vi "MainRIOJuan.vi"() -> ()   [LabVIEW 2019]
uses:
  RIOData--cluster.ctl
  Acelerometer data--cluster.ctl
  <vilib>/PantherLAB/Firebase API/PantherLAB_lib_Filtering Parameters--cluster.ctl
  a087fea8-a487-4c1c-8a8b-15f205e78756.vi
  c90b4970-0cb1-4ed8-a3e8-abf7f56642d0.vi
  079ee137-338a-4224-8d27-3950f07d8dd5.vi
  <vilib>/JDP Science/JSONtext/JSON text to Variant.vi
  <vilib>/JDP Science/JSONtext/LVClass Serializer/JSONtext LVClass Serializer.lvclass
  <vilib>/PantherLAB/Firebase API/PantherLAB_lib_firebase.lvclass
  Shared.lvlib
  <vilib>/JDP Science/JSONtext/JSONtext.lvlib
panel:
  in  "Get All":bool
  in  "Get5":bool
  out "JSON String":string
  in  "Get Newest":bool
  in  "Delete":bool
  in  "Password":string
  in  "Email":string
  in  "Log In":bool
  in  "Sign In":bool
  out "Newest":T1
  out "Data out":T1[](array[typedef])
  out "My RIO Acelerometer":T2(graph)
  # "To add an authenticated user\nto your Real Time Database"
  # "If you are already authenticated\nand you want to start using\nyour Database"
  # "Warning:\nThis button will delete all the data\nunder Post EndPoint"
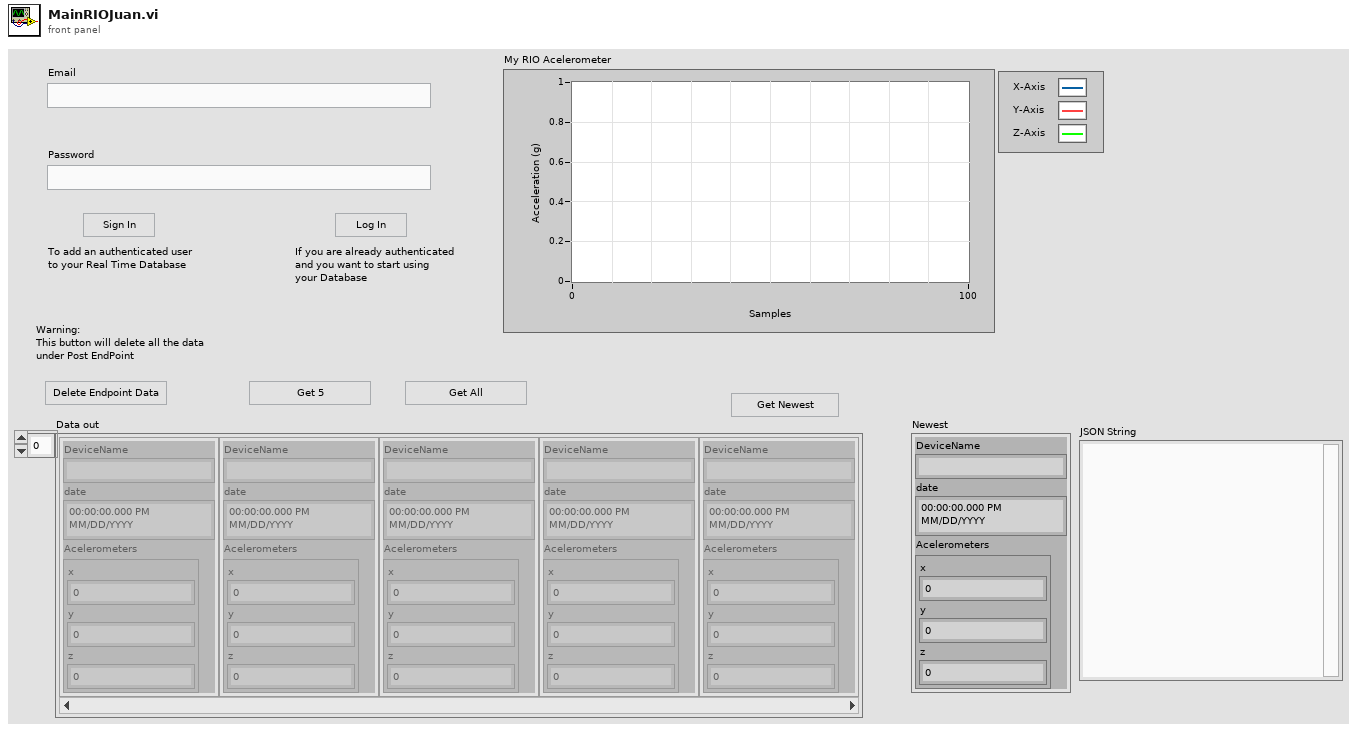
[diagram p1: front panel]
types:
  T1 = typedef "Shared.lvlib/RIOData--cluster.ctl" = cluster{"DeviceName":string, "date":timestamp, "Acelerometers":cluster{"x":dbl, "y":dbl, "z":dbl}}
  T2 = typedef "Shared.lvlib/Acelerometer data--cluster.ctl" = cluster{"X-Axis":dbl, "Y-Axis":dbl, "Z-Axis":dbl}
  T3 = cluster{"Read Access":enum8{"Allowed", "Required", "None"}, "Write Access":enum8{"Allowed", "Required", "None"}}
  T4 = typedef "PantherLAB_lib_firebase.lvclass/PantherLAB_lib_Filtering Parameters--cluster.ctl" = cluster{"Filtering Param":string, "Argument":string}
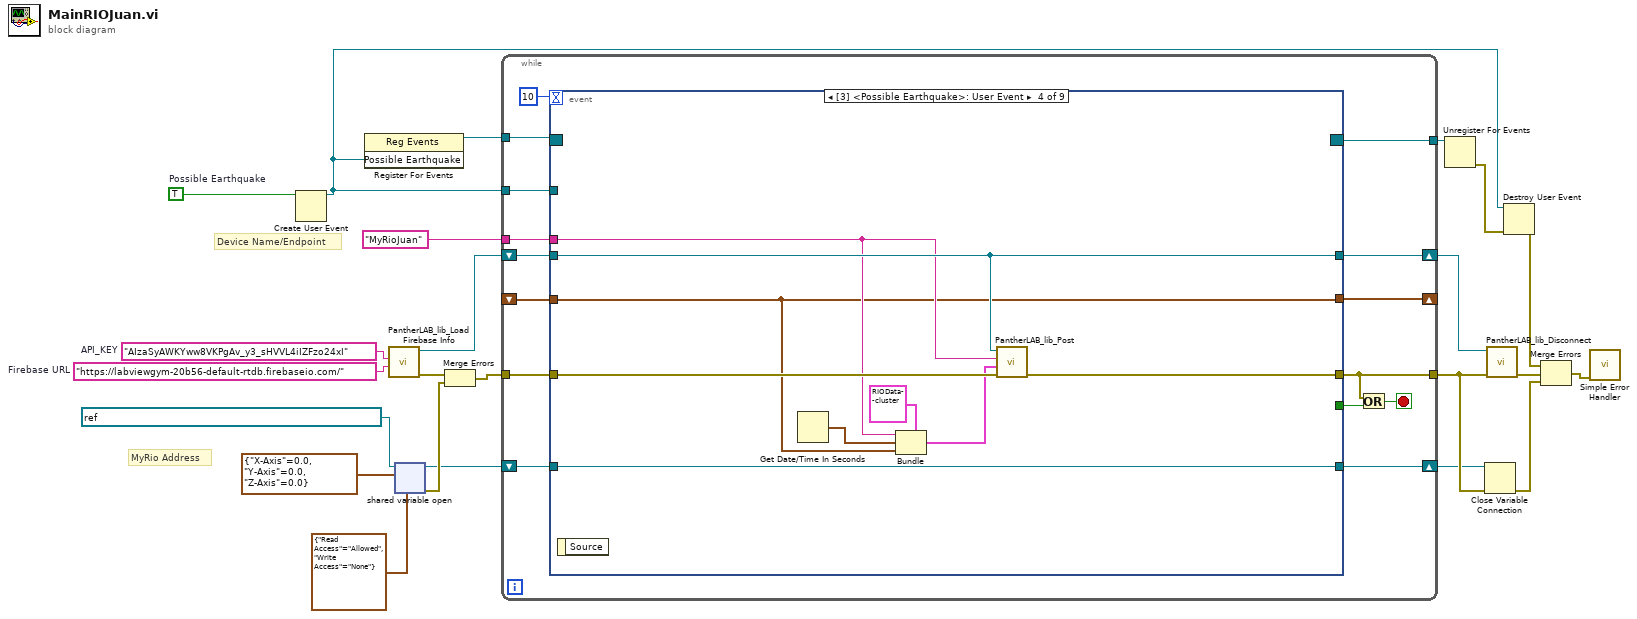
[diagram p0: block diagram]
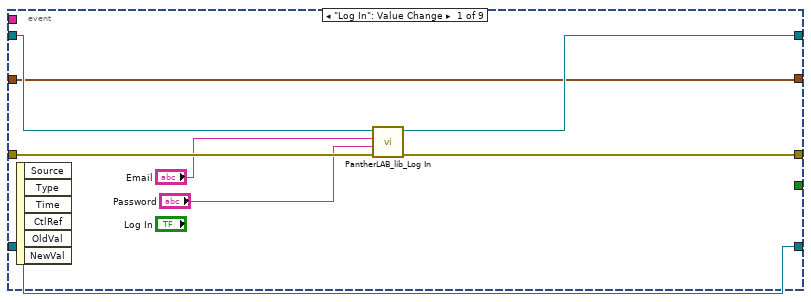
[diagram p2: hidden frame]
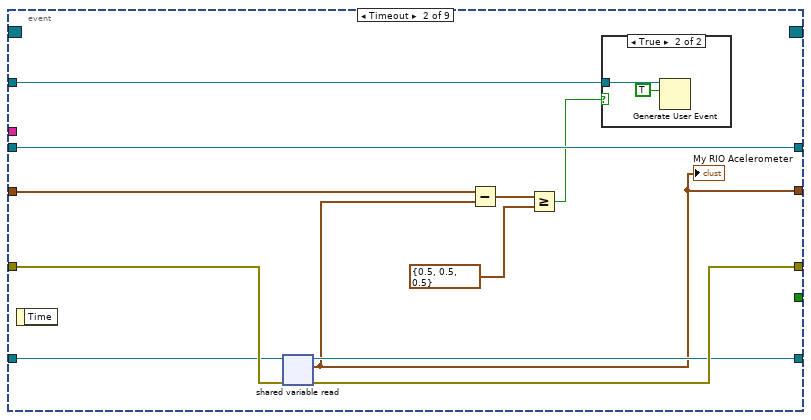
[diagram p3: hidden frame]
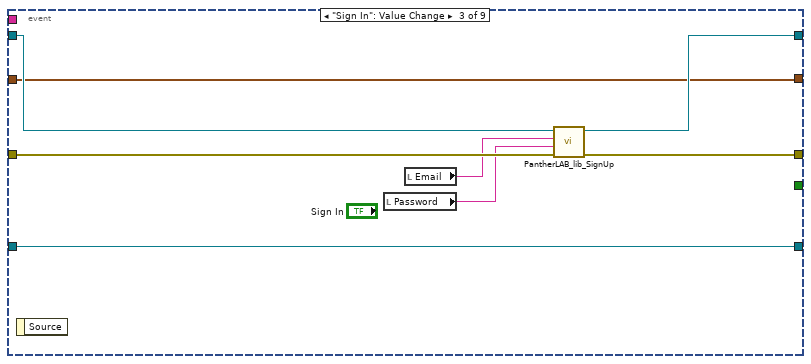
[diagram p5: hidden frame]
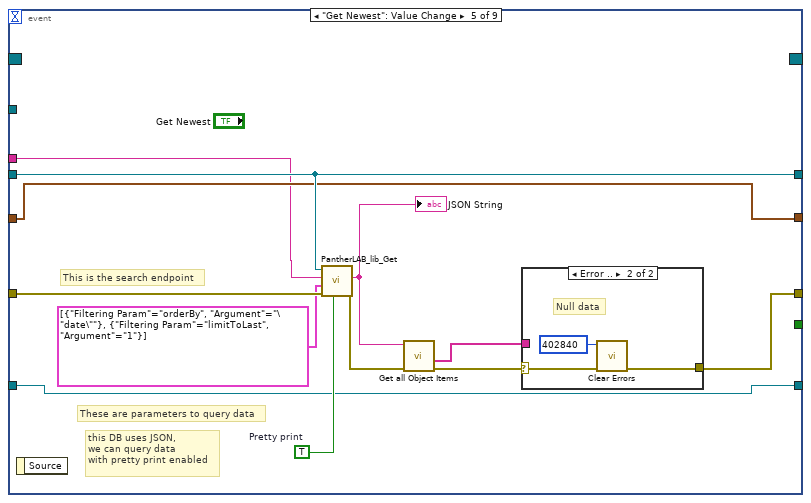
[diagram p6: hidden frame]
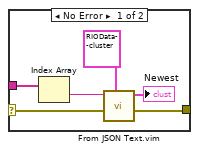
[diagram p7: hidden frame]
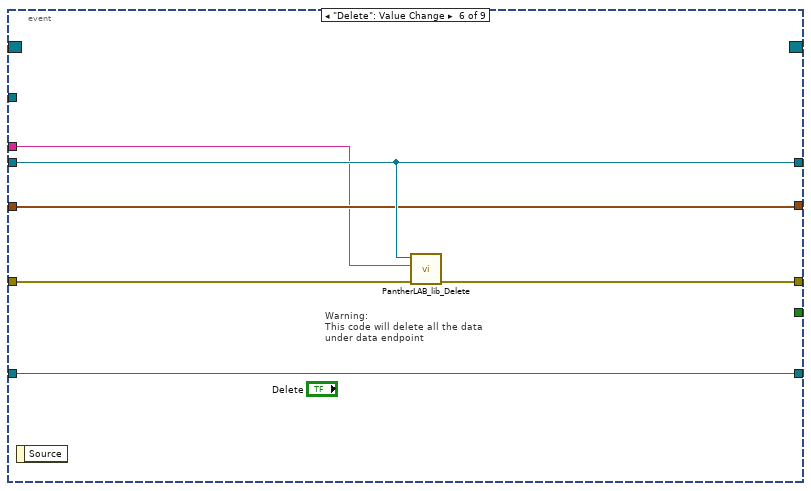
[diagram p8: hidden frame]
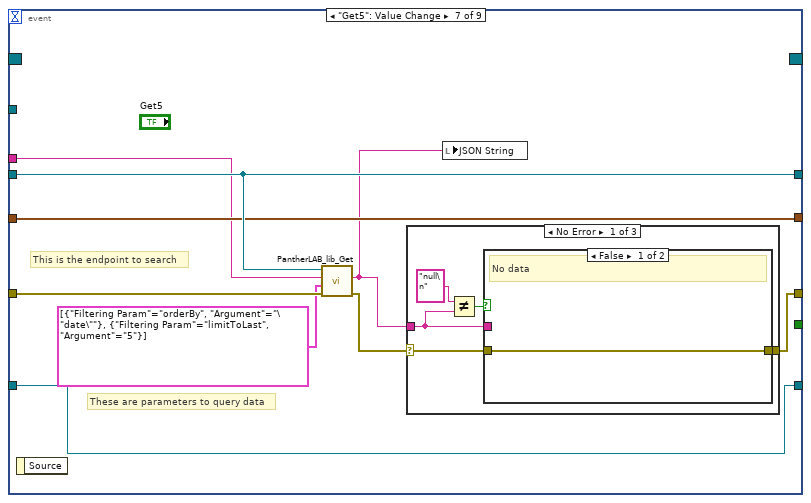
[diagram p9: hidden frame]
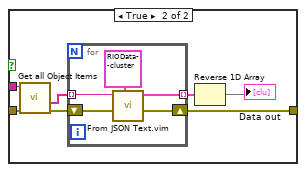
[diagram p10: hidden frame]
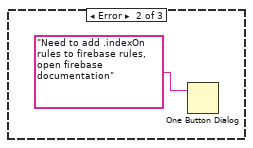
[diagram p11: hidden frame]
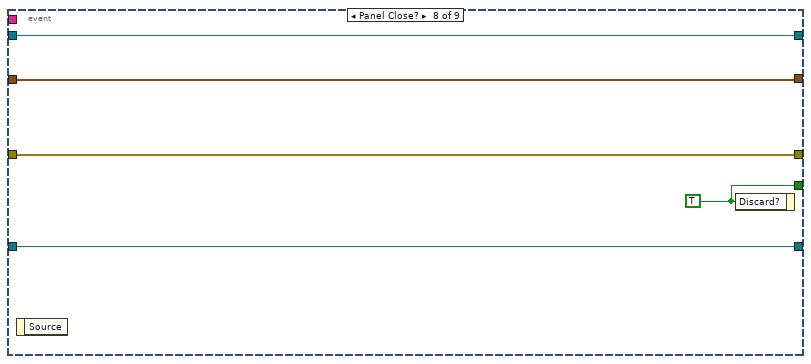
[diagram p13: hidden frame]
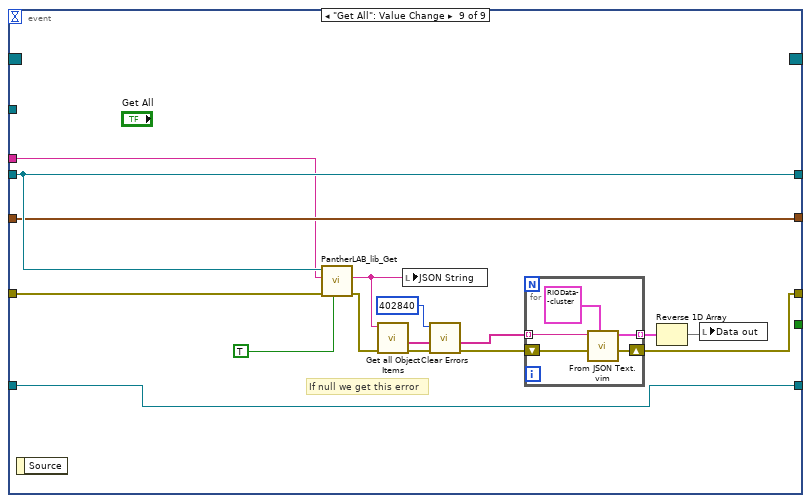
[diagram p14: hidden frame]
diagram:
  w4 = TRUE  # Possible Earthquake
  w9 = "AIzaSyAWKYww8VKPgAv_y3_sHVVL4iIZFzo24xI"  # API_KEY
  w8 = "https://labviewgym-20b56-default-rtdb.firebaseio.com/"  # Firebase URL
  # "MyRio Address"
  # "Device Name/Endpoint"
  n1 = Create User Event(user event datatype=w4) -> (user event=w2:refnum<user-event>)  [unwired: 1 in, 1 out]
  n2 = register-events(w2) -> (reference out=w5:refnum<event-registration>)  [unwired: 2 in, 1 out]
  n3 = call <vilib>:"PantherLAB_lib_Load Firebase Info.vi"("Firebase URL"=w8, "API_KEY"=w9) -> ("error out"=w22:errorcluster, "firebase out"=w10:refnum<class "PantherLAB_lib_firebase.lvclass">)  [unwired: 8 in]
  n4 = shared-variable-open(refnum<k21> "ni.var.psp://192.168.0.227/MyRioLib/AcelerationRIO" ("shared variable refnum in"), T2 {"X-Axis"=0.0, "Y-Axis"=0.0, "Z-Axis"=0.0} ("Acceleration"), T3 {"Read Access"=enum."Allowed", "Write Access"=enum."None"} ("access")) -> (w7:refnum<k21>, w20:errorcluster)  [unwired: 1 in]
  n5 = Merge Errors(w22, w20) -> (w21:errorcluster)
  n6 = while {
    tunnel: w21 -> [w38]
    tunnel: [w37] -> w19
    shift-right: [w33] -> w11
    shift-left: w10 -> [w34]
    shift-right: [w30] -> w6
    shift-left: w7 -> [w31]
    tunnel: w5 -> [w29]
    tunnel: w2 -> [w28]
    shift-right: [w27] -> _
    shift-left: _ -> [w26]
    tunnel: [w25] -> w3
    tunnel: "MyRioJuan" -> [w24]
    stop <- w35 stop-if-true
    n7 = event shown="[3] <Possible Earthquake>: User Event" {
      selector: w29 -> [_ _ _ _ _ _ _ _ _]
      dyn-events: [_ _ _ _ _ _ _ _ _] -> w25
      timeout: 10 -> [_ _ _ _ _ _ _ _ _]
      tunnel: w38 -> [w46 w57 w67 w76 w88 w103 w112 w137 w152]
      tunnel: [w45 w56 w66 w75 w86 w102 w110 w137 w149] -> w37
      tunnel: [_ _ _ _ _ _ _ w135 _] -> w36
      tunnel: w34 -> [w42 w55 w63 w74 w82 w101 w108 w136 w142]
      tunnel: [w41 w55 w62 w74 w82 w101 w108 w136 w142] -> w33
      tunnel: w31 -> [w40 w54 w61 w73 w81 w100 w107 w134 w141]
      tunnel: [w40 w53 w61 w73 w81 w100 w107 w134 w141] -> w30
      tunnel: w28 -> [_ w50 _ _ _ _ _ _ _]
      tunnel: [w39 w48 w60 w68 w80 w99 w106 w133 w140] -> w27
      tunnel: w26 -> [w39 w49 w60 w68 w80 w99 w106 w133 w140]
      tunnel: w24 -> [_ _ _ w71 w79 w98 w105 _ w139]
      event "Log In": Value Change {
        n8 = event-data() -> ()  [unwired: 1 in, 6 out]
        n9 = call-dynamic "PantherLAB_lib_Log In.vi"("error in"=w46, "password"="Password", "email"="Email", "firebase in"=w42) -> ("error out"=w45:errorcluster, "firebase out"=w41:refnum<class "PantherLAB_lib_firebase.lvclass">)  [unwired: 6 in]
      }
      event Timeout {
        n10 = event-data() -> ()  [unwired: 1 in, 1 out]
        n11 = shared-variable-read(w54, w57) -> (w53:refnum<k21>, w56:errorcluster, w48:T2)  [unwired: 1 out]
        "My RIO Acelerometer" <- w48
        n12 = Subtract(x=w49, y=w48) -> (x-y=w52:T2)
        n13 = Greater Or Equal?(x=w52, y=T2 {"X-Axis"=0.5, "Y-Axis"=0.5, "Z-Axis"=0.5} ("x")) -> (x >= y?=w47:bool)
        n14 = case shown="True" w47 {
          tunnel: w50 -> [_ w59]
          frame False {
          }
          frame True {
            n15 = Generate User Event(user event=w59, event data cluster=TRUE ("event data")) -> ()  [unwired: 2 in, 2 out]
          }
        }
      }
      event "Sign In": Value Change {
        n16 = event-data() -> ()  [unwired: 1 in, 1 out]
        n17 = local read "Password"() -> (w65:string)
        n18 = local read "Email"() -> (w64:string)
        n19 = call-dynamic "PantherLAB_lib_SignUp.vi"("error in"=w67, "password"=w65, "email"=w64, "firebase in"=w63) -> ("error out"=w66:errorcluster, "firebase out"=w62:refnum<class "PantherLAB_lib_firebase.lvclass">)  [unwired: 6 in]
      }
      event User Event {
        n20 = event-data() -> ()  [unwired: 1 in, 1 out]
        n21 = Get Date/Time In Seconds() -> (seconds since 1Jan1904=w70:timestamp)
        n22 = Bundle(cluster=T1 {"DeviceName"="", "date"=timestamp(0 s since 1904-01-01), "Acelerometers"={"x"=0.0, "y"=0.0, "z"=0.0}} ("output cluster"), "DeviceName"=w71, "date"=w70, "Acelerometers"=w68) -> (w72:T1)
        n23 = call-dynamic "PantherLAB_lib_Post.vi"("error in"=w76, "Anything"=w72, "endPoint"=w71, "firebase in"=w74) -> ("error out"=w75:errorcluster)  [unwired: 6 in, 1 out]
      }
      event "Get Newest": Value Change {
        w83 = TRUE  # Pretty print
        # "this DB uses JSON,\nwe can query data\nwith pretty print enabled"
        # "These are parameters to query data"
        # "This is the search endpoint"
        n24 = event-data() -> ()  [unwired: 1 in, 1 out]
        n25 = call-dynamic "PantherLAB_lib_Get.vi"("Pretty print"=w83, "error in"=w88, "Filtering Params"=T4[] [{"Filtering Param"="orderBy", "Argument"="\"date\""}, {"Filtering Param"="limitToLast", "Argument"="1"}], "endPoint"=w79, "firebase in"=w82) -> ("error out"=w87:errorcluster, "Json String"=w84:string)  [unwired: 5 in]
        "JSON String" <- w84
        n26 = call <vilib>:"Get all Object Items.vi"("error in (no error)"=w87, "JSON"=w84) -> ("error out"=w78:errorcluster, "<JSON>"=w77:string[])  [unwired: 6 in, 2 out]
        n27 = case shown="Error .." w78 {
          selector: w78 -> [w94 w97]
          tunnel: [w93 w96] -> w86
          tunnel: w77 -> [w92 _]
          frame No Error {
            n28 = Index Array(array=w92) -> (element=w91:string)  [unwired: 1 in]
            n29 = call "From JSON Text.vim"("Data Type and Default Value"=T1 {"DeviceName"="", "date"=timestamp(0 s since 1904-01-01), "Acelerometers"={"x"=0.0, "y"=0.0, "z"=0.0}} ("Array"), "error in (no error)"=w94, "JSON"=w91) -> ("error out"=w93:errorcluster, "Data out"=→"Newest":T1)  [unwired: 7 in]
          }
          frame Error {
            # "Null data"
            n30 = call <vilib>:"Clear Errors.vi"("error in (no error)"=w97, "specific error code to clear (0: all)"=402840) -> ("error out"=w96:errorcluster)  [unwired: 4 in, 1 out]
          }
        }
      }
      event "Delete": Value Change {
        # "Warning:\nThis code will delete all the data\nunder data endpoint"
        n31 = event-data() -> ()  [unwired: 1 in, 1 out]
        n32 = call-dynamic "PantherLAB_lib_Delete.vi"("error in"=w103, "endPoint"=w98, "firebase in"=w101) -> ("error out"=w102:errorcluster)  [unwired: 7 in, 1 out]
      }
      event "Get5": Value Change {
        # "This is the endpoint to search"
        # "These are parameters to query data"
        n33 = event-data() -> ()  [unwired: 1 in, 1 out]
        n34 = call-dynamic "PantherLAB_lib_Get.vi"("error in"=w112, "Filtering Params"=T4[] [{"Filtering Param"="orderBy", "Argument"="\"date\""}, {"Filtering Param"="limitToLast", "Argument"="5"}], "endPoint"=w105, "firebase in"=w108) -> ("error out"=w111:errorcluster, "Json String"=w104:string)  [unwired: 6 in]
        n35 = case shown="No Error" w111 {
          selector: w111 -> [w117 _ w132]
          tunnel: [w116 _ w132] -> w110
          tunnel: w104 -> [w113 _ _]
          frame No Error {
            n36 = Not Equal?(x="null\n" ("Display"), y=w113) -> (x != y?=w114:bool)
            n37 = case shown="False" w114 {
              tunnel: w117 -> [w118 w124]
              tunnel: [w118 w123] -> w116
              tunnel: w113 -> [_ w120]
              frame False {
                # "No data"
              }
              frame True {
                n38 = call <vilib>:"Get all Object Items.vi"("error in (no error)"=w124, "JSON"=w120) -> ("error out"=w125:errorcluster, "<JSON>"=w122:string[])  [unwired: 6 in, 2 out]
                n39 = for {
                  tunnel: w122 -> [w128] mode=indexing
                  shift-right: [w129] -> w123
                  shift-left: w125 -> [w130]
                  tunnel: [w127] -> w121 mode=indexing
                  n40 = call "From JSON Text.vim"("Data Type and Default Value"=T1 {"DeviceName"="", "date"=timestamp(0 s since 1904-01-01), "Acelerometers"={"x"=0.0, "y"=0.0, "z"=0.0}} ("RioData"), "error in (no error)"=w130, "JSON"=w128) -> ("error out"=w129:errorcluster, "Data out"=w127:T1)  [unwired: 7 in]
                }
                n41 = Reverse 1D Array(array=w121) -> (reversed array=→"Data out":T1[])
              }
            }
          }
          frame Error {
            n42 = One Button Dialog(message="Need to add .indexOn rules to firebase rules, open firebase documentation") -> ()  [unwired: 1 in, 1 out]
          }
          frame Default {
          }
        }
        n43 = local write "JSON String"(w104) -> ()
      }
      event Panel Close? {
        w135 = TRUE ("Discard?")
        n44 = event-data() -> ()  [unwired: 1 in, 1 out]
        n45 = event-data("Discard?"=w135) -> ()  [unwired: 1 in, 1 out]
      }
      event "Get All": Value Change {
        # "If null we get this error"
        n46 = event-data() -> ()  [unwired: 1 in, 1 out]
        n47 = call-dynamic "PantherLAB_lib_Get.vi"("Pretty print"=TRUE, "error in"=w152, "endPoint"=w139, "firebase in"=w142) -> ("error out"=w150:errorcluster, "Json String"=w145:string)  [unwired: 6 in]
        n48 = call <vilib>:"Get all Object Items.vi"("error in (no error)"=w150, "JSON"=w145) -> ("error out"=w151:errorcluster, "<JSON>"=w147:string[])  [unwired: 6 in, 2 out]
        n49 = local write "JSON String"(w145) -> ()
        n50 = call <vilib>:"Clear Errors.vi"("error in (no error)"=w151, "specific error code to clear (0: all)"=402840) -> ("error out"=w148:errorcluster)  [unwired: 4 in, 1 out]
        n51 = for {
          tunnel: w147 -> [w155] mode=indexing
          shift-right: [w156] -> w149
          shift-left: w148 -> [w157]
          tunnel: [w154] -> w146 mode=indexing
          n52 = call "From JSON Text.vim"("Data Type and Default Value"=T1 {"DeviceName"="", "date"=timestamp(0 s since 1904-01-01), "Acelerometers"={"x"=0.0, "y"=0.0, "z"=0.0}} ("RioData"), "error in (no error)"=w157, "JSON"=w155) -> ("error out"=w156:errorcluster, "Data out"=w154:T1)  [unwired: 7 in]
        }
        n53 = Reverse 1D Array(array=w146) -> (reversed array=w138:T1[])
        n54 = local write "Data out"(w138) -> ()
      }
    }
    n55 = Or(x=w37, y=w36) -> (x .or. y?=w35:bool)
  }
  n56 = Unregister For Events(event registration refnum=w3) -> (error out=w15:errorcluster)  [unwired: 1 in]
  n57 = Close Variable Connection(8:w19, 11:w6) -> (0:w17:errorcluster)
  n58 = call-dynamic "PantherLAB_lib_Disconnect.vi"("error in"=w19, "firebase in"=w11) -> ("error out"=w23:errorcluster)  [unwired: 9 in]
  n59 = Destroy User Event(user event=w2, error in=w15) -> (error out=w16:errorcluster)
  n60 = Merge Errors(w16, w23, w17) -> (w18:errorcluster)
  n61 = call <vilib>:"Simple Error Handler.vi"("error in (no error)"=w18) -> ()  [unwired: 4 in, 5 out]
